vi "Setup Radio Buttons for Dialog.vi"(6 "Show Radio":bool, 7 "Action":T1=enum."Wire Properties", 8 "error in (no error)":errorcluster, 10 "Action Choice Ref":refnum<vi>, 11 "Affected Items":T2) -> (0 "error out":errorcluster)   [LabVIEW 2023]
doc: "Radio buttons are shown for tunnels on structure with the options Inside/Outside. But for inner tunnels on a flat sequence structure, they should say Right/Left."
uses:
  top/BundleMagic.ctl
  controls/action enum.ctl
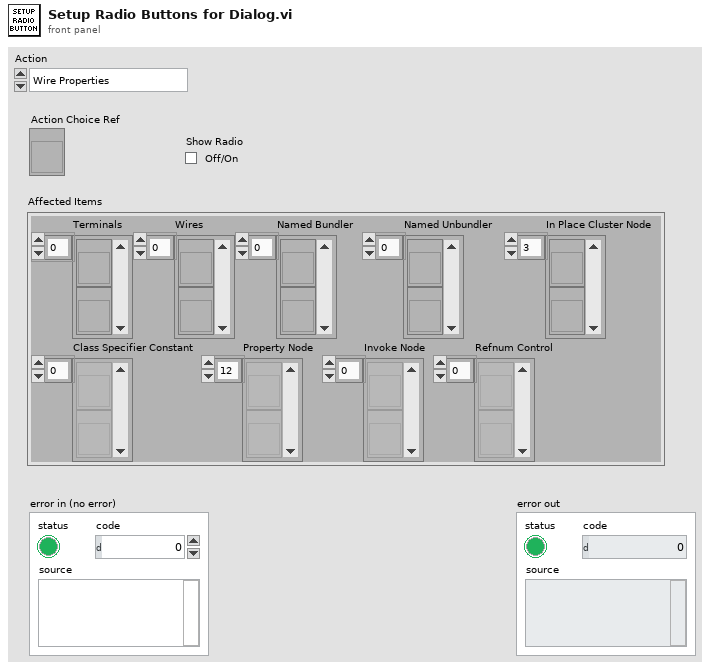
[diagram p1: front panel]
types:
  T1 = typedef "action enum.ctl" = enum16{"[NONE]", "APP_SEPARATOR", "Wire Bundle", "Wire Unbundle", "Terminal Unbundle", "Terminal Bundle", "Bundler Move Up", "Bundler Move Down", "Bundler Insert", "Bundler Remove", "Bundler Remove Unwired", "Bundler Reorder", "In Place Insert", "In Place Remove", "In Place Remove Unwired", "In Place Reorder", "Wire Properties", "Wire Method", "Terminal Properties", "Terminal Method", "Property Move Up", "Property Move Down", "Properties Insert", "Properties Remove", "Properties Remove Unwired", "Properties Reorder", "Method Change", "Class For Constant", "Class For Control", "Class For Node", "Class Name to Clipboard"}
  T2 = typedef "BundleMagic.ctl" = cluster{"Terminals":refnum<vi>[], "Wires":refnum<vi>[], "Named Bundler":refnum<vi>[], "Named Unbundler":refnum<vi>[], "In Place Cluster Node":refnum<vi>[], "Class Specifier Constant":refnum<vi>[], "Property Node":refnum<vi>[], "Invoke Node":refnum<vi>[], "Refnum Control":refnum<vi>[]}
  T3 = enum16{"[NONE]", "Wire Bundle", "Wire Unbundle", "Terminal Unbundle", "Terminal Bundle", "Bundler Insert", "Bundler Remove", "Bundler Rearrange", "In Place Insert", "In Place Remove", "In Place Rearrange", "Wire Properties", "Wire Method", "Terminal Properties", "Terminal Method", "Properties Insert", "Properties Remove", "Properties Rearrange", "Method Change", "Classes"}
  T4 = enum8{"Enabled", "Disabled", "Disabled and Grayed Out"}
  T5 = typedef "Control 1.ctl" = enum16{"Left", "Top", "Right", "Bottom"}
  T6 = cluster{"Tunnel Ref":refnum<vi>, "On Tunnel?":bool, "Placement":enum32{"Choice 1", "Choice 2"}, "Tunnel Is Indexing?":bool, "Diagram":refnum<vi>, "Position":cluster{"Refnum":refnum<vi>, "Relative Direction":enum32{"Right", "Left", "Top", "Bottom", "Top Right", "Top Left", "Bottom Right", "Bottom Left"}, "Point32":cluster{"Horizontal":i32, "Vertical":i32}}, "Chosen Terminal":refnum<vi>, "Is Refnum?":bool, "Is Cluster?":bool, "Is Source?":bool, "Tunnel Direction":enum16{"In-Going", "Out-Going"}, "Tunnel Position":T5, "Is Inner?":bool, "Terminal Is Indexing?":bool}
  T7 = enum8{"Enabled", "Disabled", "Disabled and Grayed Out"}[]
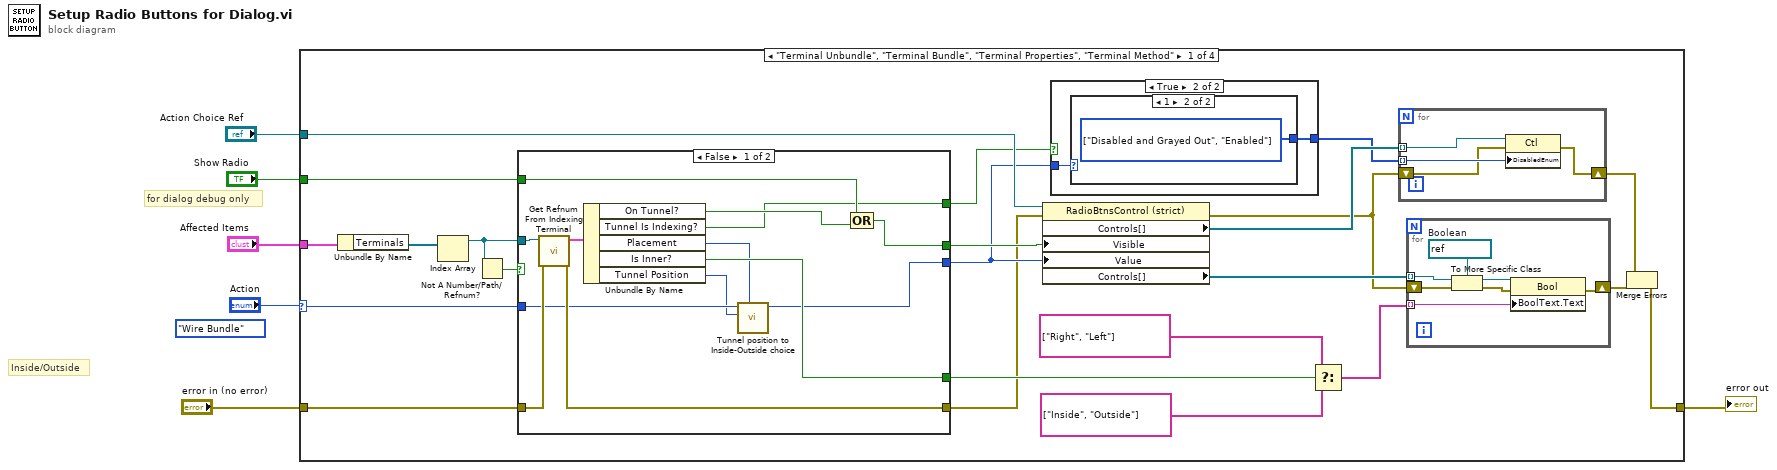
[diagram p0: block diagram]
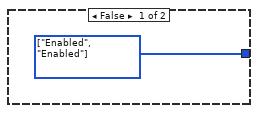
[diagram p2: hidden frame]
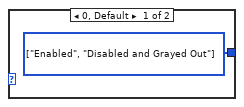
[diagram p3: hidden frame]
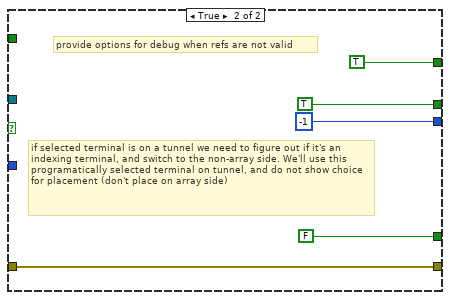
[diagram p4: hidden frame]
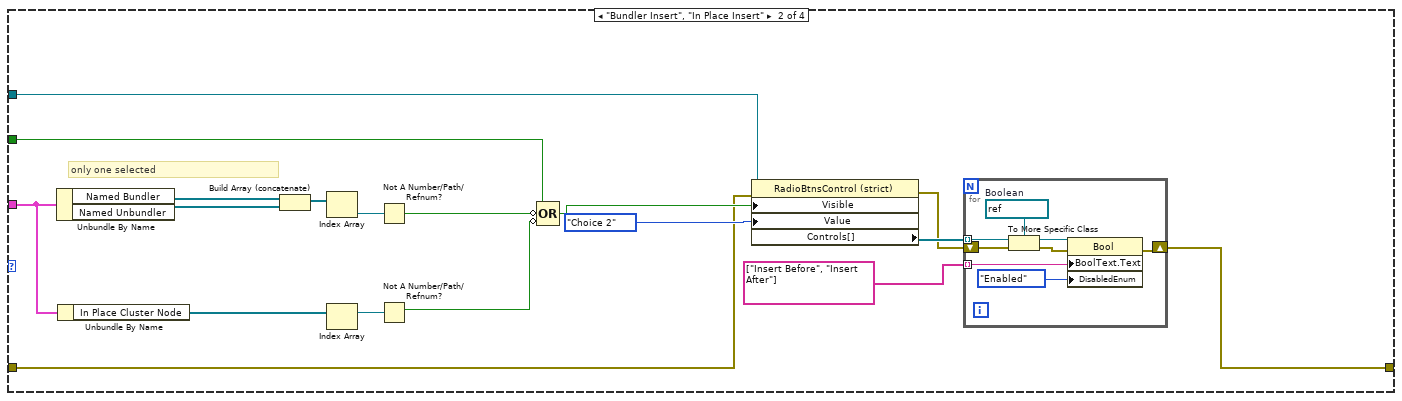
[diagram p5: hidden frame]
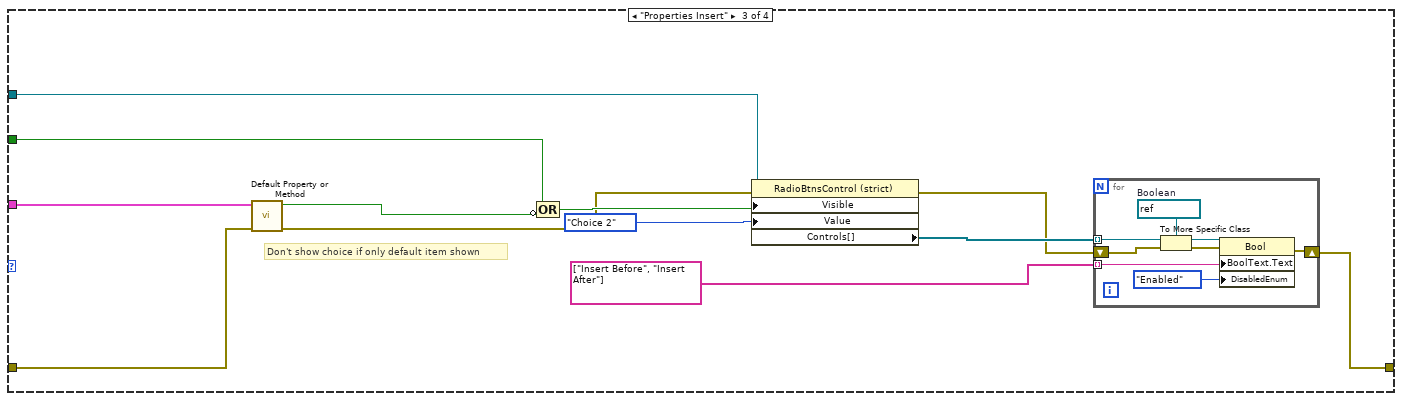
[diagram p6: hidden frame]
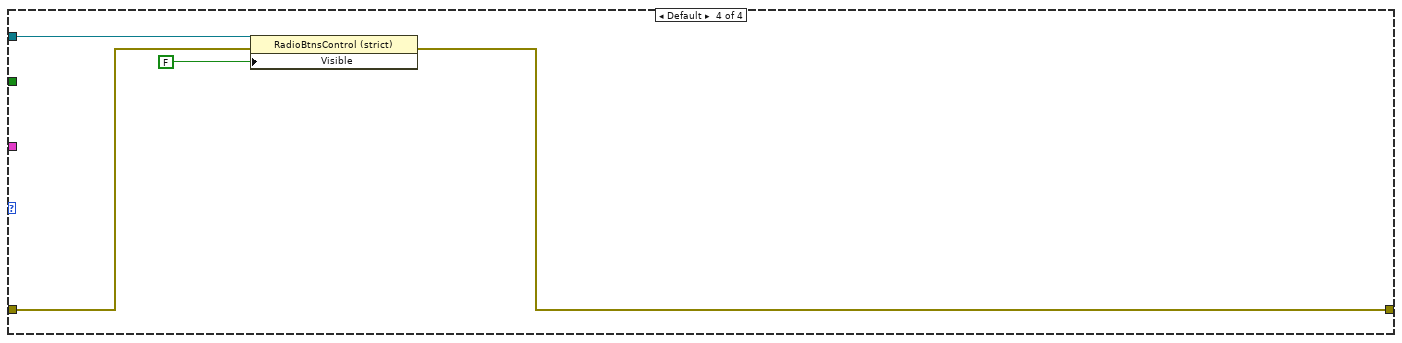
[diagram p7: hidden frame]
diagram:
  (unwired) T3."Wire Bundle" ("Action")
  # "Inside/Outside"
  # "for dialog debug only"
  n1 = case shown="\"Terminal Unbundle\", \"Terminal Bundle\", \"Terminal Properties\", \"Terminal Method\"" "Action" {
    selector: "Action" -> [w7 _ _ _]
    tunnel: "Affected Items" -> [w28 w71 w95 _]
    tunnel: "Action Choice Ref" -> [w27 w80 w101 w113]
    tunnel: "Show Radio" -> [w21 w77 w98 _]
    tunnel: "error in (no error)" -> [w13 w66 w90 w111]
    tunnel: [w8 w64 w91 w110] -> w1
    frame "Terminal Unbundle", "Terminal Bundle", "Terminal Properties", "Terminal Method" {
      n2 = Unbundle By Name(w28) -> ("Terminals"=w29:refnum<vi>[])
      n3 = Index Array(array=w29) -> (element=w19:refnum<vi>)  [unwired: 1 in]
      n4 = Not A Number/Path/Refnum?(number/path/refnum=w19) -> (NaN/Path/Refnum?=w18:bool)
      n5 = case shown="False" w18 {
        tunnel: [w51 TRUE] -> w22
        tunnel: w21 -> [w50 _]
        tunnel: w19 -> [w48 _]
        tunnel: [w40 -1] -> w14
        tunnel: [w49 FALSE] -> w20
        tunnel: [w45 TRUE ("Is Indexing?")] -> w16
        tunnel: w13 -> [w44 w52]
        tunnel: [w43 w52] -> w12
        tunnel: w7 -> [w42 _]
        frame False {
          n6 = call "Get Refnum From Indexing Terminal.vi"("error in"=w44, "Refnum Terminal"=w48) -> ("error out"=w43:errorcluster, "Terminal Data Cluster"=w47:T6)  [unwired: 6 in, 2 out]
          n7 = Unbundle By Name(w47) -> ("On Tunnel?"=w46:bool, "Tunnel Is Indexing?"=w45:bool, "Placement"=w39:enum32{"Choice 1", "Choice 2"}, "Is Inner?"=w49:bool, "Tunnel Position"=w41:T5)
          n8 = call "Tunnel position to Inside-Outside choice.vi"("Default Placement"=w39, "Tunnel Position"=w41, "Action"=w42) -> ("Placement"=w40:enum16{"Inside", "Outside"})  [unwired: 8 in]
          n9 = Compound Arithmetic op=OR(w50, w46) -> (w51:bool)
        }
        frame True {
          # "if selected terminal is on a tunnel we need to figure out if it's an indexing terminal, and switch to the non-array side. We'll use this programatically selected terminal on tunnel, and do not show choice for placement (don't place on array side)"
          # "provide options for debug when refs are not valid"
        }
      }
      n10 = property on="Property Node" class="RadioBtnsControl (strict)"(reference=w27, error in=w12, "Visible"=w22, "Value"=w14) -> (error out=w11:errorcluster, "Controls[]"=w17:refnum<vi>[], "Controls[]"=w26:refnum<vi>[])  [unwired: 1 out]
      n11 = case shown="True" w16 {
        tunnel: [w30 w31] -> w15
        tunnel: w14 -> [_ w32]
        frame False {
          w30 = T7 [enum."Enabled", enum."Enabled"] items=["Enabled", "Disabled", "Disabled and Grayed Out"] ("Disabled")
        }
        frame True {
          n12 = case shown="1" w32 {
            tunnel: [w33 w34] -> w31
            frame 0, Default {
              w33 = T7 [enum."Enabled", enum."Disabled and Grayed Out"] items=["Enabled", "Disabled", "Disabled and Grayed Out"] ("Disabled")
            }
            frame 1 {
              w34 = T7 [enum."Disabled and Grayed Out", enum."Enabled"] items=["Enabled", "Disabled", "Disabled and Grayed Out"] ("Disabled")
            }
          }
        }
      }
      n13 = Select(t=string[] ["Right", "Left"], s=w20, f=string[] ["Inside", "Outside"]) -> (s? t:f=w23:string[])
      n14 = for {
        tunnel: w17 -> [w38] mode=indexing
        tunnel: w15 -> [w37] mode=indexing
        shift-right: [w35] -> w9
        shift-left: w11 -> [w36]
        n15 = property class="Ctl"(reference=w38, error in=w36, "DisabledEnum"=w37) -> (error out=w35:errorcluster)  [unwired: 1 out]
      }
      n16 = for {
        tunnel: w26 -> [w63] mode=indexing
        tunnel: w23 -> [w62] mode=indexing
        shift-right: [w57] -> w10
        shift-left: w11 -> [w59]
        w60 = refnum<vi> refnum  # Boolean
        n17 = To More Specific Class(target class=w60, reference=w63, error in=w59) -> (specific class reference=w61:refnum<vi>, error out=w58:errorcluster)
        n18 = property on="Property Node" class="Bool"(reference=w61, error in=w58, "BoolText.Text"=w62) -> (error out=w57:errorcluster)  [unwired: 1 out]
      }
      n19 = Merge Errors(w9, w10) -> (w8:errorcluster)
    }
    frame "Bundler Insert", "In Place Insert" {
      # "only one selected"
      n20 = Unbundle By Name(w71) -> ("Named Bundler"=w76:refnum<vi>[], "Named Unbundler"=w75:refnum<vi>[])
      n21 = Unbundle By Name(w71) -> ("In Place Cluster Node"=w70:refnum<vi>[])
      n22 = Build Array (concatenate)(w76, w75) -> (w74:refnum<vi>[])
      n23 = Index Array(array=w74) -> (element=w81:refnum<vi>)  [unwired: 1 in]
      n24 = Index Array(array=w70) -> (element=w69:refnum<vi>)  [unwired: 1 in]
      n25 = Not A Number/Path/Refnum?(number/path/refnum=w81) -> (NaN/Path/Refnum?=w73:bool)
      n26 = Not A Number/Path/Refnum?(number/path/refnum=w69) -> (NaN/Path/Refnum?=w68:bool)
      n27 = Compound Arithmetic op=OR(w77, invert w73, invert w68) -> (w78:bool)
      n28 = property on="Property Node" class="RadioBtnsControl (strict)"(reference=w80, error in=w66, "Visible"=w78, "Value"=enum32{"Choice 1", "Choice 2"}."Choice 2" ("Tunnel Placement Radio Buttons")) -> (error out=w65:errorcluster, "Controls[]"=w79:refnum<vi>[])  [unwired: 1 out]
      n29 = for {
        tunnel: w79 -> [w89] mode=indexing
        tunnel: string[] ["Insert Before", "Insert After"] -> [w88] mode=indexing
        shift-right: [w82] -> w64
        shift-left: w65 -> [w84]
        w86 = refnum<vi> refnum  # Boolean
        n30 = To More Specific Class(target class=w86, reference=w89, error in=w84) -> (specific class reference=w87:refnum<vi>, error out=w83:errorcluster)
        n31 = property on="Property Node" class="Bool"(reference=w87, error in=w83, "BoolText.Text"=w88, "DisabledEnum"=T4."Enabled" ("Disabled")) -> (error out=w82:errorcluster)  [unwired: 1 out]
      }
    }
    frame "Properties Insert" {
      # "Don't show choice if only default item shown"
      n32 = call "Default Property or Method.vi"("error in"=w90, "Affected Items"=w95) -> ("error out"=w93:errorcluster, "One default element"=w94:bool)  [unwired: 8 in]
      n33 = Compound Arithmetic op=OR(w98, invert w94) -> (w99:bool)
      n34 = property on="Property Node" class="RadioBtnsControl (strict)"(reference=w101, error in=w93, "Visible"=w99, "Value"=enum32{"Choice 1", "Choice 2"}."Choice 2" ("Tunnel Placement Radio Buttons")) -> (error out=w92:errorcluster, "Controls[]"=w100:refnum<vi>[])  [unwired: 1 out]
      n35 = for {
        tunnel: w100 -> [w109] mode=indexing
        tunnel: string[] ["Insert Before", "Insert After"] -> [w108] mode=indexing
        shift-right: [w102] -> w91
        shift-left: w92 -> [w104]
        w106 = refnum<vi> refnum  # Boolean
        n36 = To More Specific Class(target class=w106, reference=w109, error in=w104) -> (specific class reference=w107:refnum<vi>, error out=w103:errorcluster)
        n37 = property on="Property Node" class="Bool"(reference=w107, error in=w103, "BoolText.Text"=w108, "DisabledEnum"=T4."Enabled" ("Disabled")) -> (error out=w102:errorcluster)  [unwired: 1 out]
      }
    }
    frame Default {
      n38 = property on="Property Node" class="RadioBtnsControl (strict)"(reference=w113, error in=w111, "Visible"=FALSE) -> (error out=w110:errorcluster)  [unwired: 1 out]
    }
  }
  "error out" <- w1
